vi "Delete (array).vi"(8 "error in (no error)":errorcluster, 10 "Path Array":string[](array[string]), 11 "JSON Value in":refnum<class "JSON Value.lvclass">) -> (0 "error out":errorcluster, 3 "JSON Value out":refnum<class "JSON Value.lvclass">)   [LabVIEW 2017, in "JSON Value.lvclass"]
uses:
  JSON Value.lvclass
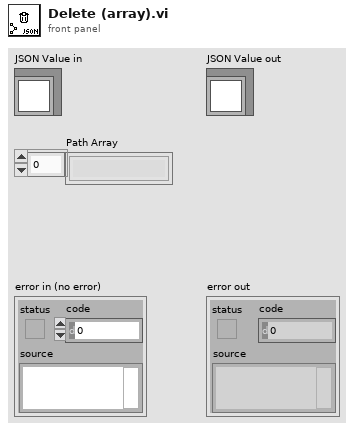
[diagram p1: front panel]
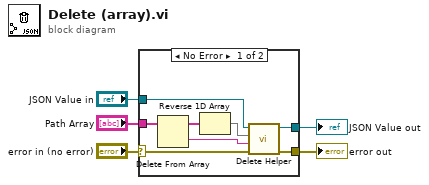
[diagram p0: block diagram]
diagram:
  n1 = case shown="No Error" "error in (no error)" {
    selector: "error in (no error)" -> [w12 w14]
    tunnel: [w10 w15] -> w3
    tunnel: "JSON Value in" -> [w13 w15]
    tunnel: "Path Array" -> [w8 _]
    tunnel: [w9 w14] -> w1
    frame No Error {
      n2 = Delete From Array(array=w8) -> (deleted portion=w6:string, array with subset deleted=w7:string[])  [unwired: 2 in]
      n3 = Reverse 1D Array(array=w7) -> (reversed array=w11:string[])
      n4 = call "Delete Helper.vi"("error in (no error)"=w12, "last key"=w6, "Array"=w11, "JSON Value in"=w13) -> ("error out"=w9:errorcluster, "JSON Value out"=w10:refnum<class "JSON Value.lvclass">)  [unwired: 6 in]
    }
    frame Error {
    }
  }
  "error out" <- w1
  "JSON Value out" <- w3
